vi "Encode Pulse Count.vi"(1 "Pulse count":i16) -> (0 "Array":u8[](array[numeric]) format="%x")   [LabVIEW 2013]
panel:
  # "Return data to write for pulse count, including start address"
  # "Address"
  # "MSB"
  # "LSB"
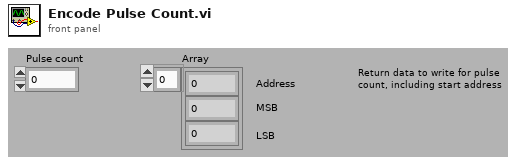
[diagram p1: front panel]
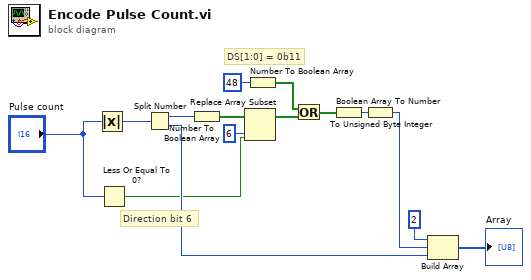
[diagram p0: block diagram]
diagram:
  # "DS[1:0] = 0b11"
  # "Direction bit 6"
  n1 = Absolute Value(x="Pulse count") -> (abs(x)=w9:i16)
  n2 = Less Or Equal To 0?(x="Pulse count") -> (x <= 0?=w13:bool)
  n3 = Split Number(x=w9) -> (hi(x)=w10:u8, lo(x)=w14:u8)
  n4 = Number To Boolean Array(number=w10) -> (Boolean array=w11:bool[])
  n5 = Replace Array Subset(array=w11, new element=w13, index=6) -> (w4:bool[])
  n6 = Number To Boolean Array(number=u8 48 ("lo(x)")) -> (Boolean array=w2:bool[])
  n7 = Or(x=w2, y=w4) -> (x .or. y?=w3:bool[])
  n8 = Boolean Array To Number(Boolean array=w3) -> (number=w7:u32)
  n9 = To Unsigned Byte Integer(number=w7) -> (unsigned 8bit integer=w6:u8)
  n10 = Build Array(u8 2 ("lo(x)"), w6, w14) -> (→"Array":u8[])
